vi "Create Canvas.vi"(8 "error in (no error)":errorcluster, 9 "Z":sgl, 10 "Y":sgl, 11 "X":sgl) -> (0 "error out":errorcluster, 3 "SceneObject out":refnum<vi>)   [LabVIEW 2020]
doc: "This VI creates the canvas box SceneObject that represents the sample."
uses:
  <vilib>/picture/3D Picture Control/Object/Create Object (drawable).vi
  <vilib>/picture/3D Picture Control/NI_3D Picture Control.lvlib
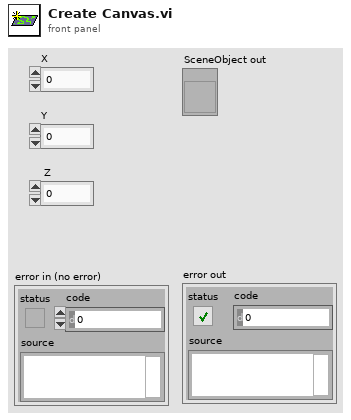
[diagram p1: front panel]
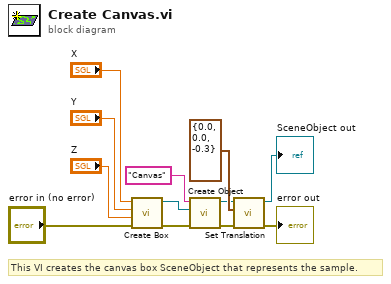
[diagram p0: block diagram]
diagram:
  # "This VI creates the canvas box SceneObject that represents the sample."
  n1 = call <vilib>:"Create Box.vi"("error in (no error)"="error in (no error)", "Length Z"="Z", "Length Y"="Y", "Length X"="X") -> ("error out"=w12:errorcluster, "New Box Refnum"=w11:refnum<vi>)  [unwired: 6 in]
  n2 = call-poly <vilib>:"Create Object.vi"("error in (no error)"=w12, "Geometry"=w11, "Name"="Canvas") -> ("error out"=w1:errorcluster, "Scene:New Object"=w4:refnum<vi>)  [unwired: 7 in]
  n3 = call <vilib>:"Set Translation.vi"("error in (no error)"=w1, "Translation"=cluster{"X":dbl, "Y":dbl, "Z":dbl} {"X"=0.0, "Y"=0.0, "Z"=-0.3} ("offset"), "Scene Object"=w4) -> ("error out"=→"error out":errorcluster, "Translated Object"=→"SceneObject out":refnum<vi>)  [unwired: 7 in]
